vi "CheckSummCalc (SubVI).vi"(11 "String in":string) -> (3 "CheckSumm_U32":u32)   [LabVIEW 2017, in "LV_Unicorn.lvlib"]
uses:
  LV_Unicorn.lvlib
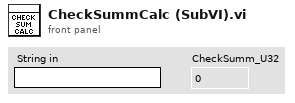
[diagram p1: front panel]
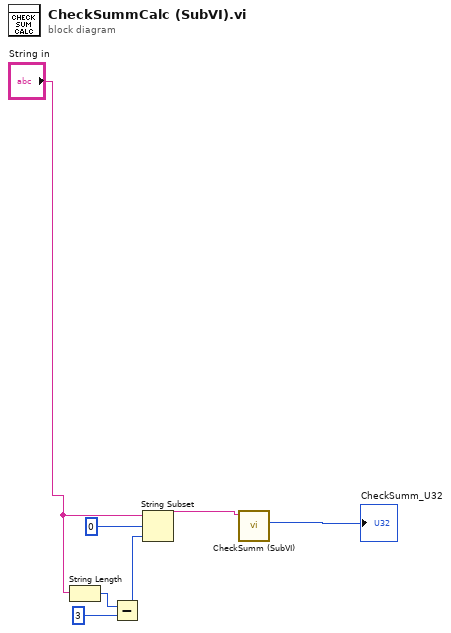
[diagram p0: block diagram]
diagram:
  n1 = String Length(string="String in") -> (length=w5:i32)
  n2 = Subtract(x=w5, y=3) -> (x-y=w7:i32)
  n3 = String Subset(string="String in", offset (0)=0, length (rest)=w7) -> (substring=w3:string)
  n4 = call "CheckSumm (SubVI).vi"("Input String"=w3) -> ("CheckSumm_U32"=→"CheckSumm_U32":u32)  [unwired: 7 in, 3 out]
